vi "Snapshot to String.vi"(7 "format string":string="Test Details: \"%s\"\nSelected Test: %s\n\nTested w/Ver. %s,\n\nSet Points:\nStep Height:, %s\nRange:, %s\nRPM:, %s\nRES:, %s\nLoad Bank:, %s\n\nMeasurments:\nSnapshot,Date,Time,Step Height,Range,RPM,RES,Load,Torque (in*lb),RPM,%s%s", 8 "error in":errorcluster, 11 "Snapshot":T1={"Test Details"="", "Version"="test", "Date"=timestamp(0 s since 1904-01-01), "Selected Test"="", "Snapshot Number"=0, "Time"=timestamp(0 s since 1904-01-01), "Ibrake Setpoint"="", "RPM Setpoint"="", "Range Setpoint"="", "Step Height Setpoint"="", "Load Bank Setpoint"="", "Measurement Headers"="", "Measurements"="", "A"=0, "B"=0, "C"=0, "Raw Data"=[], "Available Tests"=enum."Manual", "Ibrake List"="", "RPM List"="", "Load Bank List"="", "Range List"="", "Step Height List"="", "FanMode Setpoint"=enum."Auto"} {"Time" format="%<%H:%M:%S>T"; "Date" format="%<%m/%d/%Y>T"}) -> (0 "error out":errorcluster, 2 "Measurements":string, 3 "Headers and Measurements":string)   [LabVIEW 2017]
uses:
  Controls/Snapshot Typedef.ctl
  Controls/Available Tests.ctl
  Controls/FanMode.ctl
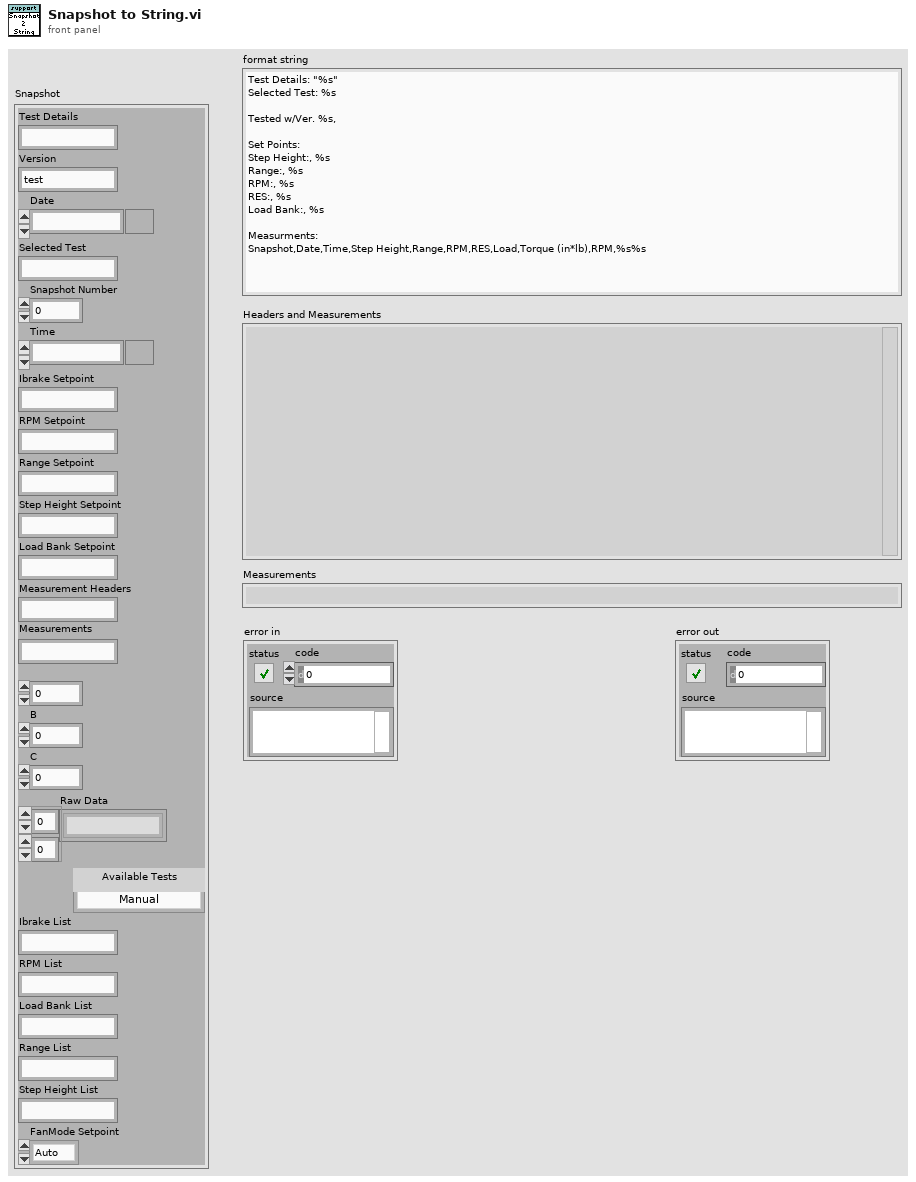
[diagram p1: front panel]
types:
  T1 = typedef "Snapshot Typedef.ctl" = cluster{"Test Details":string, "Version":string, "Date":timestamp, "Selected Test":string, "Snapshot Number":u16, "Time":timestamp, "Ibrake Setpoint":string, "RPM Setpoint":string, "Range Setpoint":string, "Step Height Setpoint":string, "Load Bank Setpoint":string, "Measurement Headers":string, "Measurements":string, "A":i32, "B":i32, "C":i32, "Raw Data":string[][], "Available Tests":T2, "Ibrake List":string, "RPM List":string, "Load Bank List":string, "Range List":string, "Step Height List":string, "FanMode Setpoint":T3}
  T2 = typedef "Available Tests.ctl" = enum16{"Manual", "EFX Brake Torque", "Generator Torque", "EFX Brake Thermal", "Generator Thermal", "Pulsed RPM", "AMT Brake Torque", "Bike Brake Torque", "AMT Brake Thermal", "Bike Brake Thermal"}
  T3 = typedef "FanMode.ctl" = enum16{"On", "Off", "Auto"}
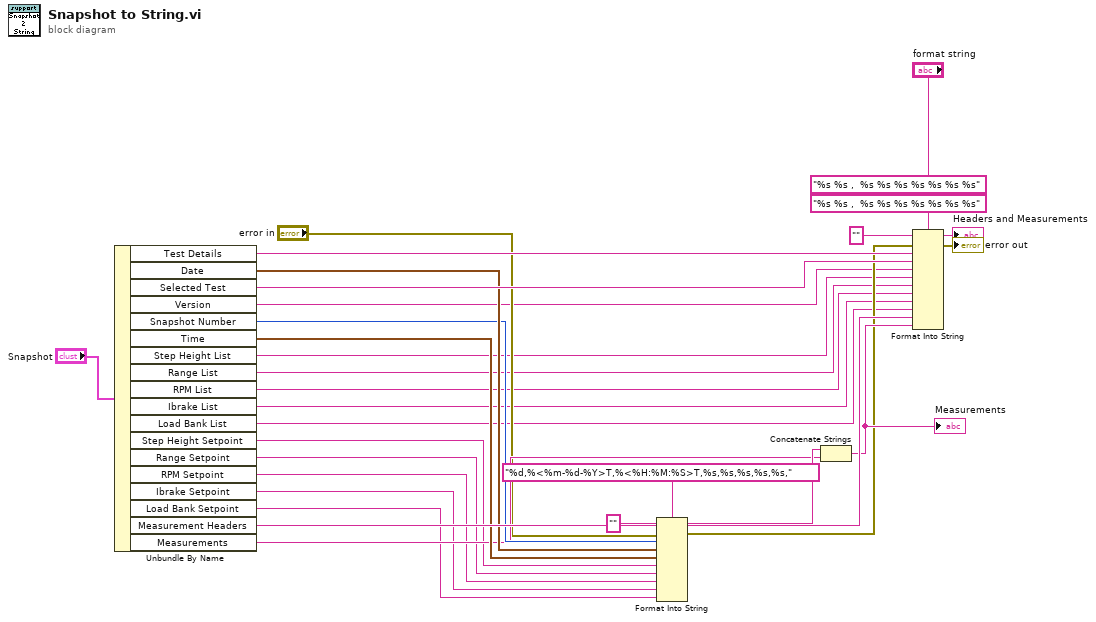
[diagram p0: block diagram]
diagram:
  (unwired) "%s %s ,  %s %s %s %s %s %s %s" ("format string")
  (unwired) "%s %s ,  %s %s %s %s %s %s %s" ("format string")
  n1 = Unbundle By Name("Snapshot") -> ("Test Details"=w27:string, "Date"=w20:timestamp, "Selected Test"=w26:string, "Version"=w1:string, "Snapshot Number"=w18:u16, "Time"=w19:timestamp, "Step Height List"=w11:string, "Range List"=w10:string, "RPM List"=w3:string, "Ibrake List"=w2:string, "Load Bank List"=w9:string, "Step Height Setpoint"=w8:string, "Range Setpoint"=w7:string, "RPM Setpoint"=w6:string, "Ibrake Setpoint"=w5:string, "Load Bank Setpoint"=w4:string, "Measurement Headers"=w25:string, "Measurements"=w16:string)
  n2 = Format Into String(format string="%d,%<%m-%d-%Y>T,%<%H:%M:%S>T,%s,%s,%s,%s,%s,", initial string="", error in="error in", w18, w20, w19, w8, w7, w6, w5, w4) -> (resulting string=w17:string, error out=w12:errorcluster)
  n3 = Concatenate Strings(w17, w16) -> (w15:string)
  "Measurements" <- w15
  n4 = Format Into String(format string="format string", initial string="", error in=w12, w27, w26, w1, w11, w10, w3, w2, w9, w25, w15) -> (resulting string=→"Headers and Measurements":string, error out=→"error out":errorcluster)
